vi "N_forsed_bitsB.vi"(3 "IN":bool[](array[boolean])) -> (1 "N_forsed_bits":i32)   [LabVIEW 2019, in "Logik.lvlib"]
uses:
  Logik.lvlib
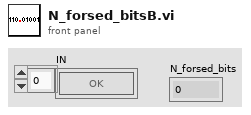
[diagram p1: front panel]
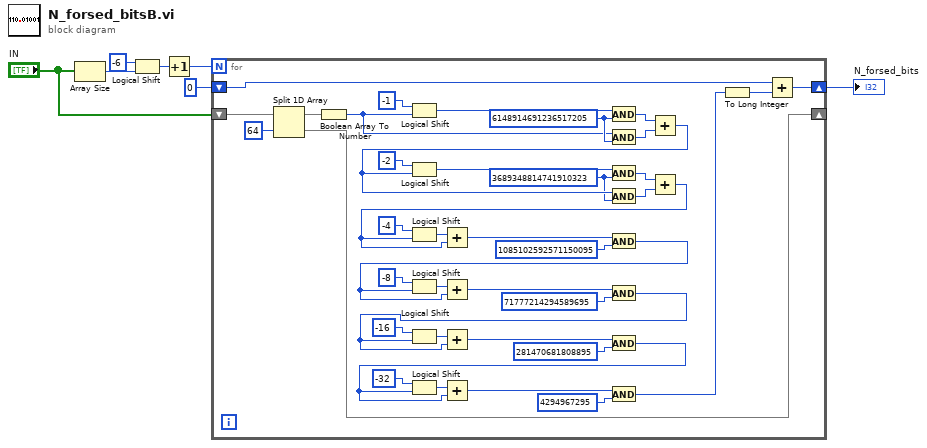
[diagram p0: block diagram]
diagram:
  n1 = Array Size(array="IN") -> (size(s)=w6:i32)
  n2 = Logical Shift(y=i16 -6, x=w6) -> (x << y=w4:i32)
  n3 = Increment(x=w4) -> (x+1=w3:i32)
  n4 = for {
    N: w3 -> [_]
    shift-right: [w46] -> w2
    shift-left: 0 -> [w45]
    shift-right: [w41] -> _
    shift-left: "IN" -> [w43]
    w18 = u64 3689348814741910323 ("y")
    w15 = u64 6148914691236517205 ("y")
    n5 = Split 1D Array(array=w43, index=64 ("length")) -> (first subarray=w42:bool[], second subarray=w41:bool[])
    n6 = Boolean Array To Number(Boolean array=w42) -> (number=w9:u64)
    n7 = Logical Shift(y=i16 -1, x=w9) -> (x << y=w21:u64)
    n8 = And(x=w21, y=w15) -> (x .and. y?=w16:u64)
    n9 = And(x=w9, y=w15) -> (x .and. y?=w17:u64)
    n10 = Add(x=w16, y=w17) -> (x+y=w25:u64)
    n11 = Logical Shift(y=i16 -2, x=w25) -> (x << y=w24:u64)
    n12 = And(x=w24, y=w18) -> (x .and. y?=w19:u64)
    n13 = And(x=w25, y=w18) -> (x .and. y?=w20:u64)
    n14 = Add(x=w19, y=w20) -> (x+y=w28:u64)
    n15 = Logical Shift(y=i16 -4, x=w28) -> (x << y=w27:u64)
    n16 = Add(x=w27, y=w28) -> (x+y=w29:u64)
    n17 = And(x=w29, y=u64 1085102592571150095) -> (x .and. y?=w38:u64)
    n18 = Logical Shift(y=i16 -8, x=w38) -> (x << y=w33:u64)
    n19 = Add(x=w33, y=w38) -> (x+y=w32:u64)
    n20 = And(x=w32, y=u64 71777214294589695) -> (x .and. y?=w39:u64)
    n21 = Logical Shift(y=i16 -16, x=w39) -> (x << y=w35:u64)
    n22 = Add(x=w35, y=w39) -> (x+y=w36:u64)
    n23 = And(x=w36, y=u64 281470681808895) -> (x .and. y?=w11:u64)
    n24 = Logical Shift(y=i16 -32, x=w11) -> (x << y=w14:u64)
    n25 = Add(x=w14, y=w11) -> (x+y=w13:u64)
    n26 = And(x=w13, y=u64 4294967295) -> (x .and. y?=w8:u64)
    n27 = To Long Integer(number=w8) -> (32bit integer=w47:i32)
    n28 = Add(x=w45, y=w47) -> (x+y=w46:i32)
  }
  "N_forsed_bits" <- w2
